vi "Material-Line3-Aquisition.vi"(8 "error in (no error)":errorcluster, 11 "Material-RunTest in":refnum<class "Material-RunTest.lvclass">) -> (0 "error out":errorcluster, 3 "Material-RunTest out":refnum<class "Material-RunTest.lvclass">)   [LabVIEW 2013, in "Material-RunTest.lvclass"]
uses:
  Material-RunTest.lvclass
  Material-RunTest.lvclass/Material-RunTest.ctl
  <instrlib>/Keyence LK-G5000/Public/enum/LKIF_OUTNO.ctl
  <vilib>/Utility/file.llb/Write To Spreadsheet File (DBL).vi
  <instrlib>/Keyence LK-G5000/Keyence LK-G5000.lvlib
  Motion Control/Motion-ControlAll.lvclass
  <vilib>/addons/_LabVIEW Style Book/Utilities/Style Book Utilities.lvlib
panel:
  out "Laser Value":sgl format="%_6g"
  out "Init Meas1":dbl[](array[numeric])
  out "stop collecting":bool=TRUE
  out "Meas 1 Dyn Data":dbl[](graph)
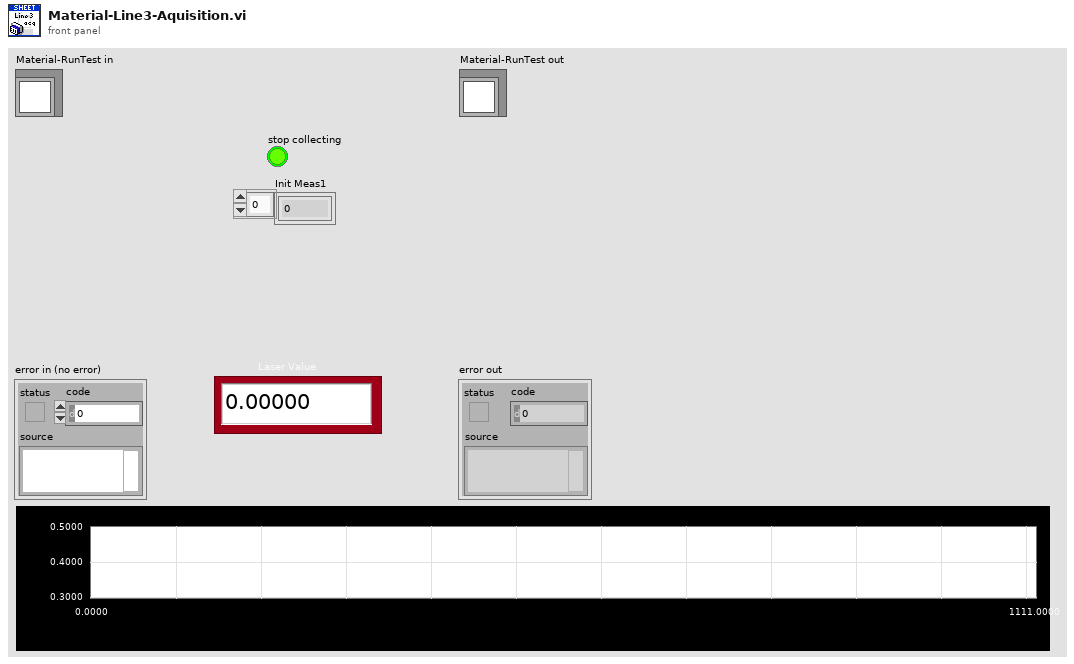
[diagram p1: front panel]
types:
  T1 = typedef "Keyence LK-G5000.lvlib/LKIF_OUTNO.ctl" = i32
  T2 = typedef "Keyence LK-G5000.lvlib/LKIF_FLOATRESULT.ctl" = i32
  T3 = cluster{"OutNo":i32, "LKIF_FLOATRESULT":T2, "Value":sgl}[]
  T4 = cluster{"OutNo":i32, "LKIF_FLOATRESULT":T2, "Value":sgl}
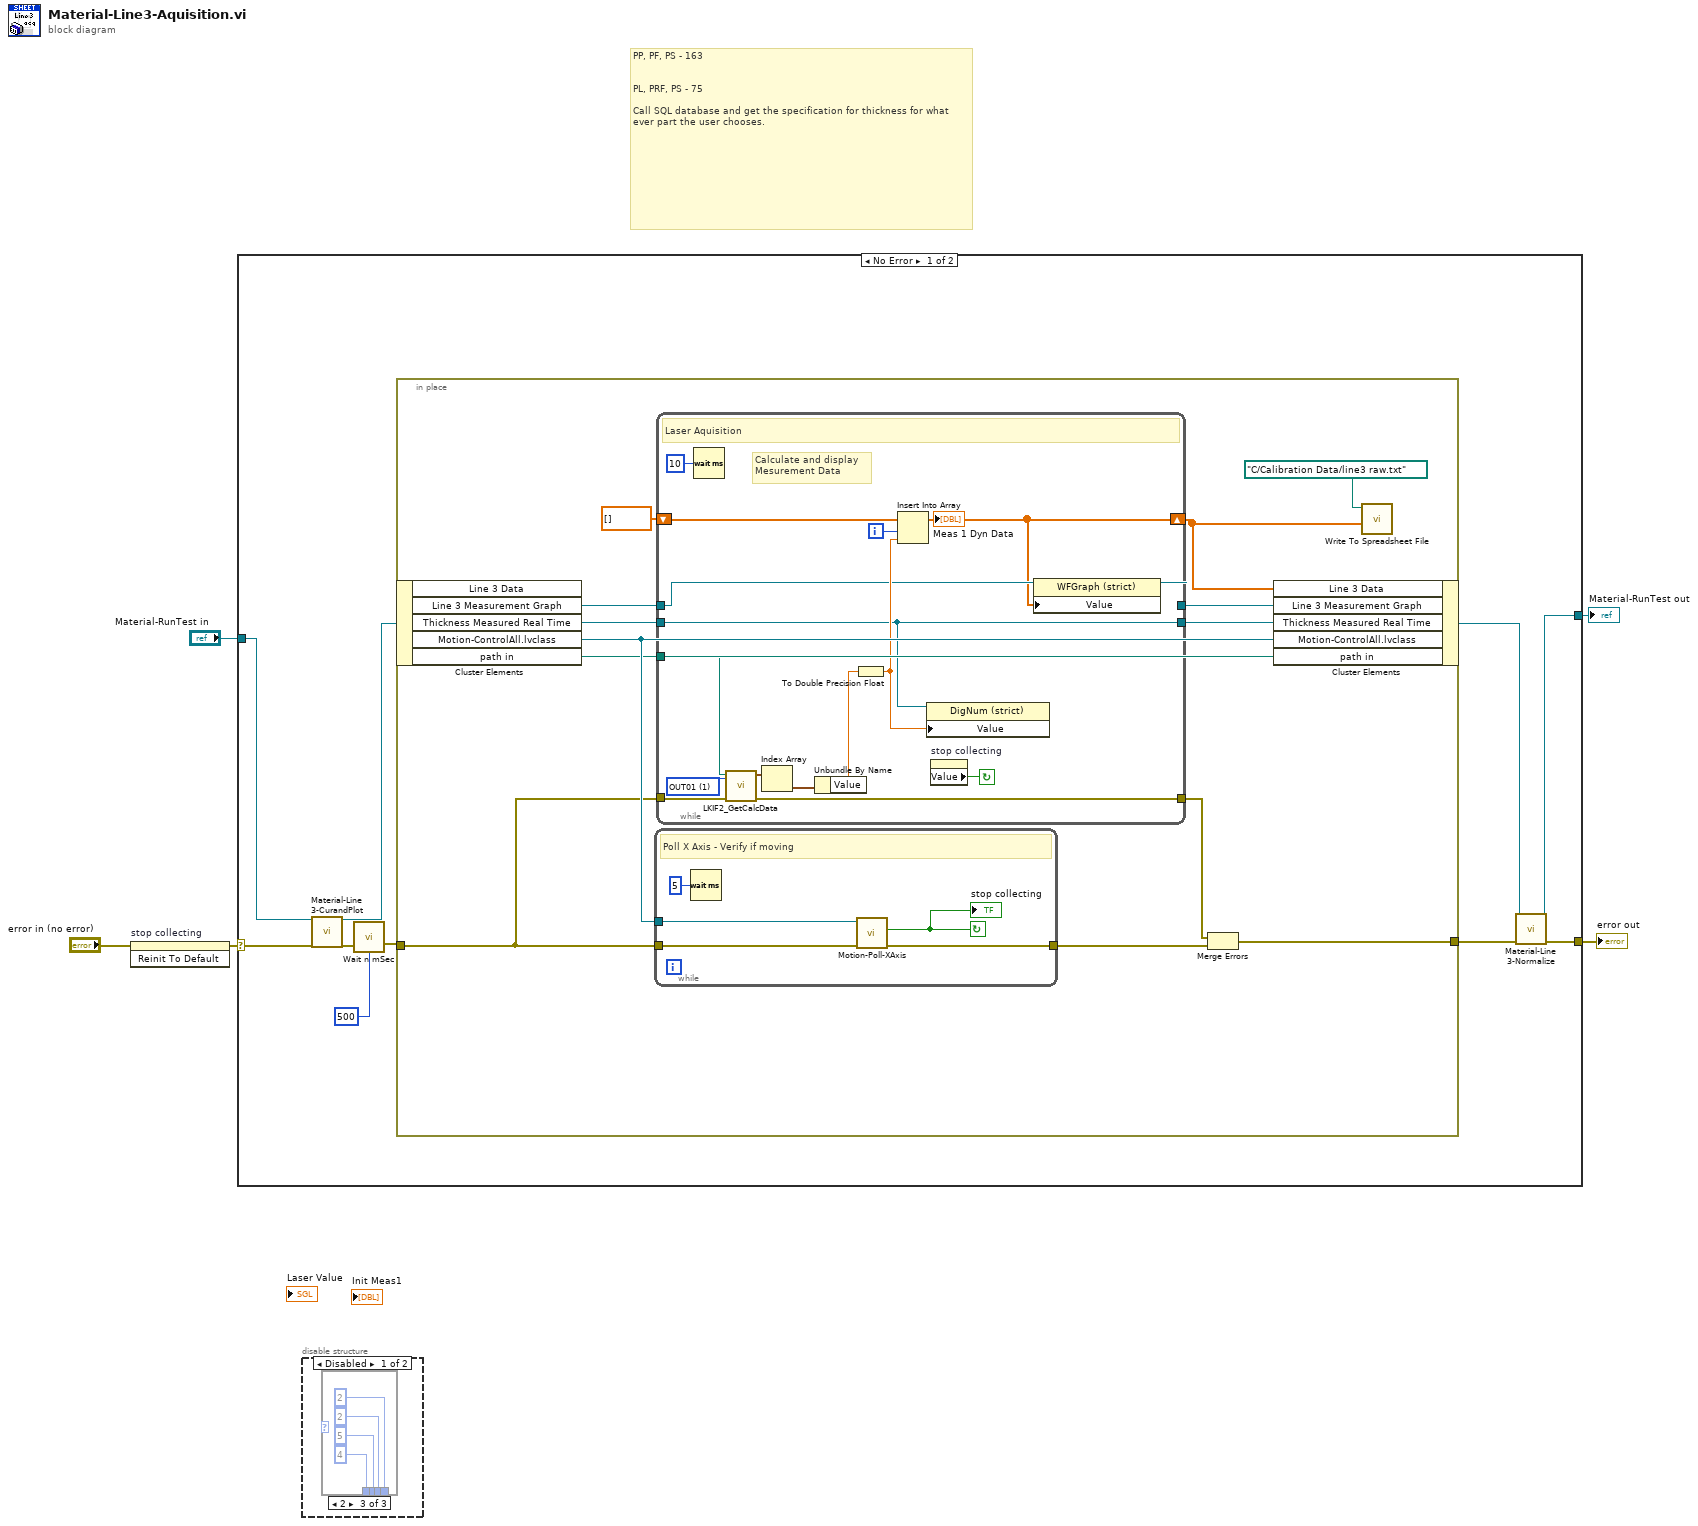
[diagram p0: block diagram]
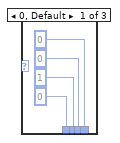
[diagram p2: hidden frame]
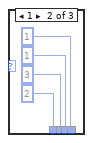
[diagram p3: hidden frame]
diagram:
  # "PP, PF, PS - 163\n\n\nPL, PRF, PS - 75\n\nCall SQL database and get the specification for thickness for what ever part the user chooses."
  n1 = invoke on="stop collecting" class="Bool (strict)" method="Reinit To Default"(error in="error in (no error)") -> (error out=w2:errorcluster)  [unwired: 2 in, 2 out]
  n2 = case shown="No Error" w2 {
    selector: w2 -> [w14 w51]
    tunnel: [w9 w51] -> w5
    tunnel: [w10 w50] -> w3
    tunnel: "Material-RunTest in" -> [w15 w50]
    frame No Error {
      n3 = call "Material-Line 3-CurandPlot.vi"("Material-RunTest in"=w15, "error in (no error)"=w14) -> ("Material-RunTest out"=w13:refnum<class "Material-RunTest.lvclass">, "error out"=w7:errorcluster)  [unwired: 16 in]
      n4 = call <vilib>:"Wait n mSec.vi"("error in (no error)"=w7, "Milliseconds to Wait (500)"=u32 500) -> ("error out"=w6:errorcluster)  [unwired: 13 in]
      n5 = in-place {
        in-place-border: w6 -> [w16]
        in-place-border: [w23] -> w12
        n6 = in-place-cluster #1(w13) -> ("Line 3 Measurement Graph"=w22:refnum<vi>, "Thickness Measured Real Time"=w27:refnum<vi>, "Motion-ControlAll.lvclass"=w26:refnum<class "Motion-ControlAll.lvclass">, "path in"=w17:path)  [unwired: 1 out]
        n7 = while {
          tunnel: w16 -> [w32]
          tunnel: [w30] -> w25
          tunnel: w26 -> [w31]
          stop <- w29 continue-if-true
          # "Poll X Axis - Verify if moving"
          n8 = Wait (ms)(milliseconds to wait=u32 5) -> ()  [unwired: 1 out]
          n9 = call "Motion-Poll-XAxis.vi"("error in (no error)"=w32, "Motion-ControlAll in"=w31) -> ("error out"=w30:errorcluster, "X axis \nstopped"=w29:bool)  [unwired: 7 in, 1 out]
          "stop collecting" <- w29
        }
        n10 = while {
          tunnel: w16 -> [w49]
          tunnel: [w45] -> w24
          shift-right: [w37] -> w18
          shift-left: dbl[] [] -> [w43]
          tunnel: w27 -> [w35]
          tunnel: w22 -> [w38]
          tunnel: [w36] -> w21
          tunnel: [w35] -> w20
          tunnel: w17 -> [w34]
          i -> [w42]
          stop <- w41 continue-if-true
          w48 = T1 1 items=["OUT01"=1, "OUT02"=2, "OUT03"=4, "OUT04"=8, "OUT05"=16, "OUT06"=32, "OUT07"=64, "OUT08"=128, "OUT09"=256, "OUT10"=512, "OUT11"=1024, "OUT12"=2048, "ALL OUT"=4095] ("OutNo (OUT1)")
          # "Calculate and display \nMesurement Data"
          # "Laser Aquisition"
          n11 = Wait (ms)(milliseconds to wait=u32 10) -> ()  [unwired: 1 out]
          n12 = call <instrlib>:"LKIF2_GetCalcData.vi"("OutNo (OUT1)"=w48, "error in (no error)"=w49, "path in"=w34) -> ("error out"=w45:errorcluster, "CalcData"=w47:T3)  [unwired: 7 in]
          n13 = Index Array(array=w47) -> (element=w46:T4)  [unwired: 1 in]
          n14 = Unbundle By Name(w46) -> ("Value"=w40:sgl)
          n15 = To Double Precision Float(number=w40) -> (double precision float=w39:dbl)
          n16 = Insert Into Array(array=w43, index=w42, new element=w39) -> (w37:dbl[])
          "Meas 1 Dyn Data" <- w37
          n17 = property class="DigNum (strict)"(reference=w35, "Value"=w39) -> ()  [unwired: 1 in, 2 out]
          n18 = property on="stop collecting" class="Bool (strict)"() -> ("Value"=w41:bool)  [unwired: 2 in, 2 out]
          n19 = property class="WFGraph (strict)"(reference=w38, "Value"=w37) -> (reference out=w36:refnum<vi>)  [unwired: 1 in, 1 out]
        }
        n20 = Merge Errors(w24, w25) -> (w23:errorcluster)
        n21 = in-place-cluster #1("Line 3 Data"=w18, "Line 3 Measurement Graph"=w21, "Thickness Measured Real Time"=w20, "Motion-ControlAll.lvclass"=w26, "path in"=w17) -> (w11:refnum<class "Material-RunTest.lvclass">)
        n22 = call-poly <vilib>:"Write To Spreadsheet File.vi"("1D data"=w18, "file path (dialog if empty)"=path "C:/Calibration Data/line3 raw.txt") -> ()  [unwired: 6 in, 1 out]
      }
      n23 = call "Material-Line 3-Normalize.vi"("error in (no error)"=w12, "Material-RunTest in"=w11) -> ("error out"=w9:errorcluster, "Material-RunTest out"=w10:refnum<class "Material-RunTest.lvclass">)  [unwired: 8 in]
    }
    frame Error {
    }
  }
  "error out" <- w5
  "Material-RunTest out" <- w3
  n24 = disable-structure shown="Disabled" {
    frame Disabled {
      n25 = case shown="2" {
        selector: _ -> [_ _ _]
        tunnel: [u32 0 ("Active Cursor Max") u32 2 ("Active Cursor Max") u32 4 ("Active Cursor Max")] -> _
        tunnel: [u32 1 ("Active Cursor Min") u32 3 ("Active Cursor Min") u32 5 ("Active Cursor Min")] -> _
        tunnel: [0 ("Active Y Scale") 1 ("Active Y Scale") 2 ("Active Y Scale")] -> _
        tunnel: [u32 0 ("Active Plot") u32 1 ("Active Plot") u32 2 ("Active Plot")] -> _
        frame 0, Default {
        }
        frame 1 {
        }
        frame 2 {
        }
      }
    }
    frame Enabled {
    }
  }
